vi "LvIRKit_InpuButtonName_Panel.vi"() -> (1 "buttunName":string, 2 "Cancel?":bool)   [LabVIEW 2014]
panel:
  in  "Button":string(combo)="電源" caption="ボタン"
  in  "Type":string(combo)="TV" caption="機器"
  in  "Place":string(combo)="リビング" caption="場所"
  out "name":string caption="登録名"
  in  "Btn Cancel":bool
  in  "Btn OK":bool
  # "ボタンの名前を入力してください"
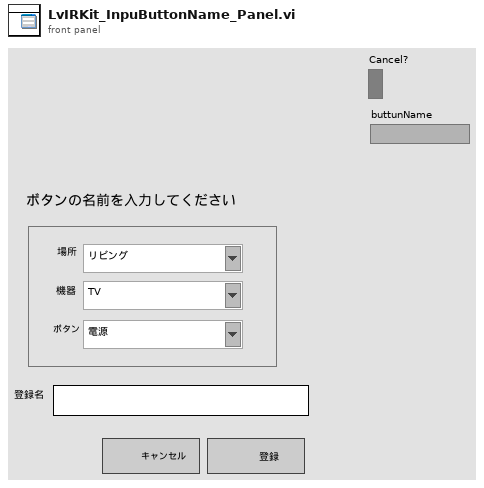
[diagram p1: front panel]
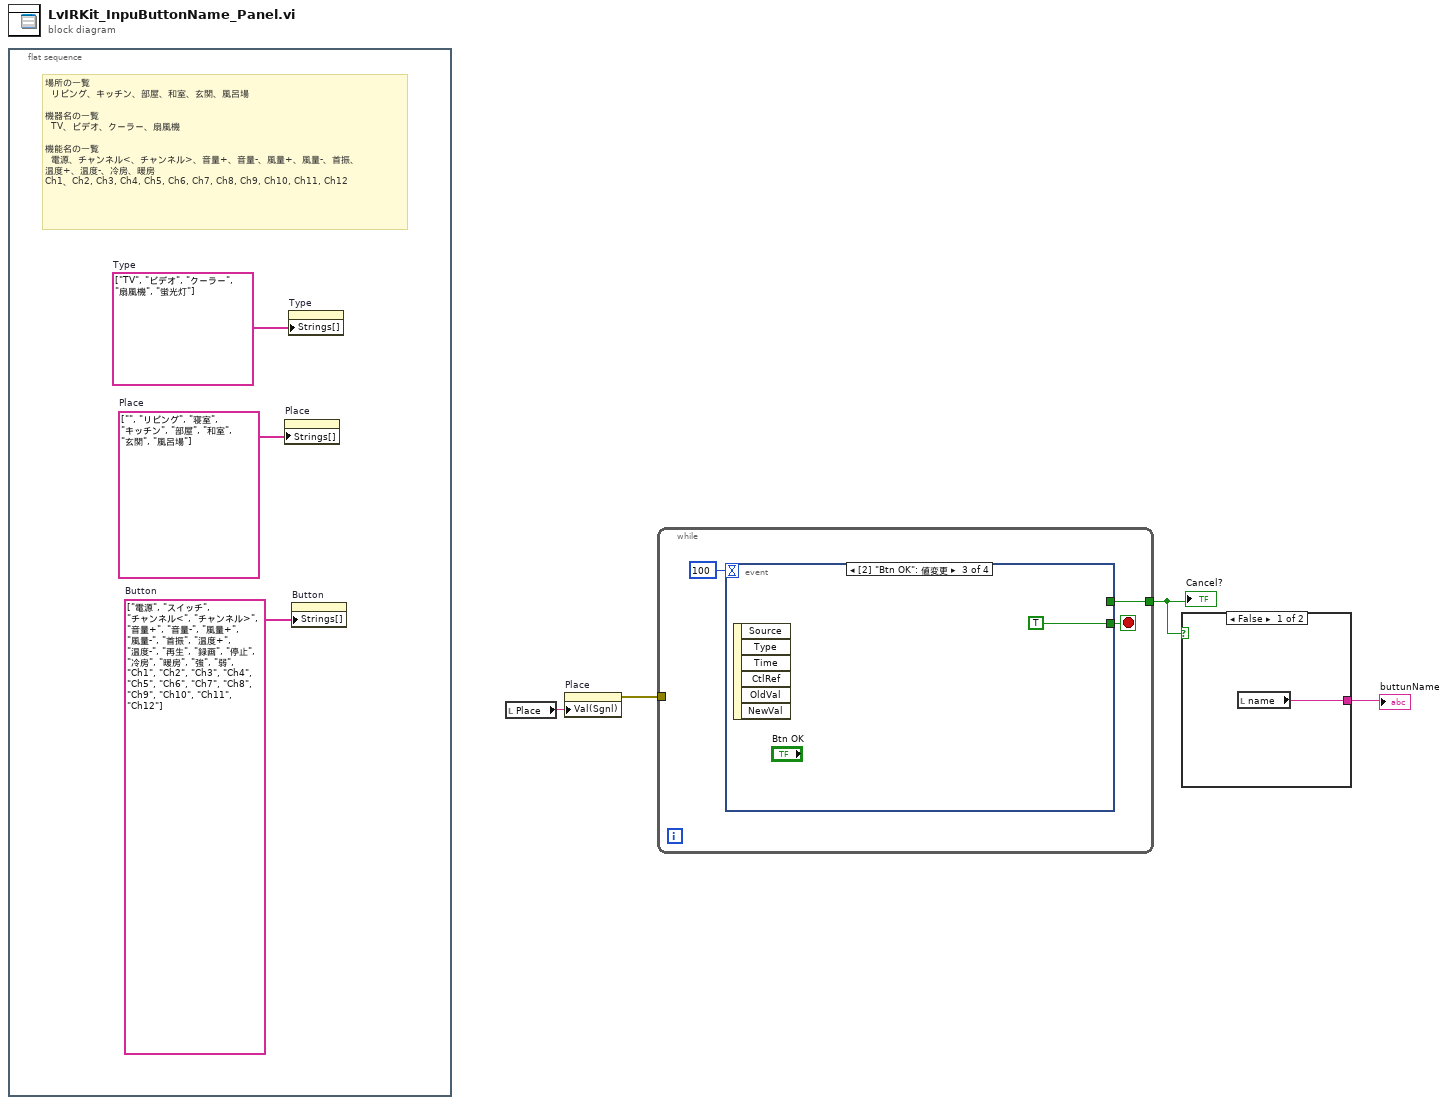
[diagram p0: block diagram]
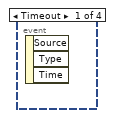
[diagram p3: hidden frame]
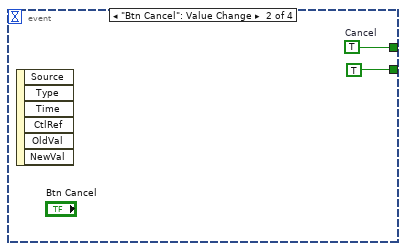
[diagram p4: hidden frame]
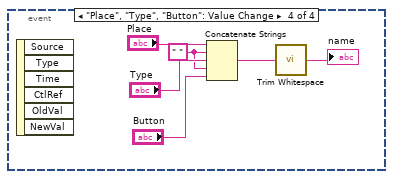
[diagram p5: hidden frame]
diagram:
  n1 = flat-sequence {
    frame #0 {
      w5 = string[] ["電源", "スイッチ", "チャンネル<", "チャンネル>", "音量+", "音量-", "風量+", "風量-", "首振", "温度+", "温度-", "再生", "録画", "停止", "冷房", "暖房", "強", "弱", "Ch1", "Ch2", "Ch3", "Ch4", "Ch5", "Ch6", "Ch7", "Ch8", "Ch9", "Ch10", "Ch11", "Ch12"]  # Button
      w6 = string[] ["", "リビング", "寝室", "キッチン", "部屋", "和室", "玄関", "風呂場"]  # Place
      w7 = string[] ["TV", "ビデオ", "クーラー", "扇風機", "蛍光灯"]  # Type
      # "場所の一覧\n  リビング、キッチン、部屋、和室、玄関、風呂場\n\n機器名の一覧\n  TV、ビデオ、クーラー、扇風機\n\n機能名の一覧\n  電源、チャンネル<、チャンネル>、音量+、音量-、風量+、風量-、首振、\n温度+、温度-、冷房、暖房\nCh1、Ch2, Ch3, Ch4, Ch5, Ch6, Ch7, Ch8, Ch9, Ch10, Ch11, Ch12"
      n2 = property on="Place" class="CmbBox"("Strings[]"=w6) -> ()  [unwired: 2 in, 2 out]
      n3 = property on="Type" class="CmbBox"("Strings[]"=w7) -> ()  [unwired: 2 in, 2 out]
      n4 = property on="Button" class="CmbBox"("Strings[]"=w5) -> ()  [unwired: 2 in, 2 out]
    }
  }
  n5 = local read "Place"() -> (w4:string)
  n6 = property on="Place" class="CmbBox"("Val(Sgnl)"=w4) -> (error out=w3:errorcluster)  [unwired: 2 in, 1 out]
  n7 = while {
    tunnel: w3 -> [_]
    tunnel: [w8] -> w1
    stop <- w9 stop-if-true
    n8 = event shown="[2] \"Btn OK\": 値変更" {
      selector: _ -> [_ _ _ _]
      dyn-events: _ -> [_ _ _ _]
      timeout: 100 -> [_ _ _ _]
      tunnel: [_ TRUE TRUE _] -> w9
      tunnel: [_ w11 _ _] -> w8
      event Timeout {
        n9 = event-data() -> ()  [unwired: 1 in, 3 out]
      }
      event "Btn Cancel": Value Change {
        w11 = TRUE  # Cancel
        n10 = event-data() -> ()  [unwired: 1 in, 6 out]
      }
      event "Btn OK": Value Change {
        n11 = event-data() -> ()  [unwired: 1 in, 6 out]
      }
      event "Place", "Type", "Button": Value Change {
        w15 = " " ("文字列")
        n12 = event-data() -> ()  [unwired: 1 in, 6 out]
        n13 = Concatenate Strings("Place", w15, "Type", w15, "Button") -> (w19:string)
        n14 = call <vilib>:"Trim Whitespace.vi"("string"=w19) -> ("trimmed string"=→"name":string)  [unwired: 1 in]
      }
    }
  }
  "Cancel?" <- w1
  n15 = case shown="FALSE" w1 {
    tunnel: [w20 _] -> w2
    frame False {
      n16 = local read "name"() -> (w20:string)
    }
    frame True {
    }
  }
  "buttunName" <- w2
